vi "emi_Text from App Version.vi"(2 "Version Info":T1={"Name"="NA", "Major"=0, "Minor"=0, "Fix"=0, "Build"=0, "Type"=enum."Alfa", "Dev"=FALSE, "Version Name"="", "Date"=timestamp(0 s since 1904-01-01)} {"Date" format="%<%y%m%d>T"}, 5 "error in (no error)":errorcluster) -> (10 "Version Name":string, 11 "DEV Text":string, 12 "Name":string, 13 "Dev Only Version":bool, 14 "Filename string":string, 15 "Short version":string, 16 "Short version Type":string, 17 "Long version":string, 18 "Full version":string, 19 "error out":errorcluster)   [LabVIEW 2011]
uses:
  Private/emi_Version Info.ctl
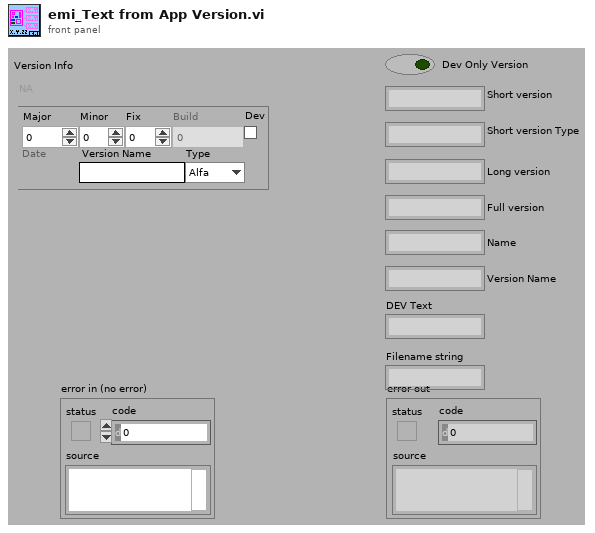
[diagram p1: front panel]
types:
  T1 = typedef "emi_Version Info.ctl" = cluster{"Name":string, "Major":i16, "Minor":i16, "Fix":i16, "Build":i32, "Type":enum16{"Alfa", "Beta", "Stable"}, "Dev":bool, "Version Name":string, "Date":timestamp}
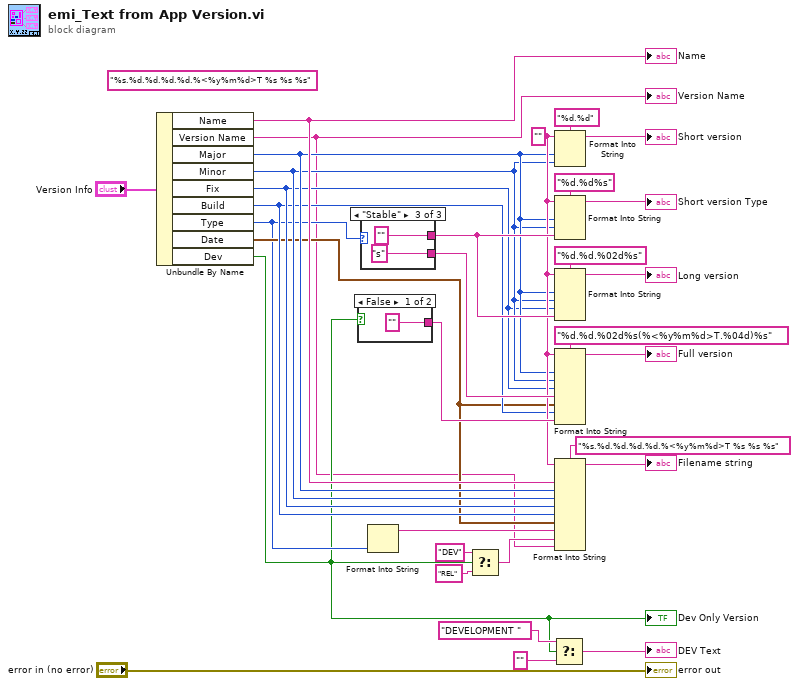
[diagram p0: block diagram]
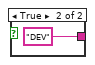
[diagram p2: hidden frame]
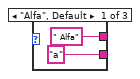
[diagram p3: hidden frame]
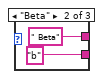
[diagram p4: hidden frame]
diagram:
  (unwired) "%s.%d.%d.%d.%d.%<%y%m%d>T %s %s %s" ("format string")
  w14 = "" ("initial string")
  n1 = Unbundle By Name("Version Info") -> ("Name"=w15:string, "Version Name"=w2:string, "Major"=w13:i16, "Minor"=w12:i16, "Fix"=w11:i16, "Build"=w10:i32, "Type"=w8:enum16{"Alfa", "Beta", "Stable"}, "Date"=w9:timestamp, "Dev"=w4:bool)
  "Dev Only Version" <- w4
  "Name" <- w15
  "Version Name" <- w2
  n2 = case shown="False" w4 {
    tunnel: ["" "DEV"] -> w29
    frame False {
      (unwired) ""
    }
    frame True {
    }
  }
  n3 = case shown="\"Stable\"" w8 {
    tunnel: [" Alfa" " Beta" ""] -> w21
    tunnel: ["a" "b" "s"] -> w27
    frame "Alfa", Default {
    }
    frame "Beta" {
    }
    frame "Stable" {
    }
  }
  n4 = Format Into String(w8) -> (resulting string=w7:string)  [unwired: 3 in, 1 out]
  n5 = Select(t="DEV" ("Version Name"), s=w4, f="REL") -> (s? t:f=w3:string)
  n6 = Select(t="DEVELOPMENT " ("Version Short"), s=w4, f="") -> (s? t:f=→"DEV Text":string)
  n7 = Format Into String(format string="%d.%d", initial string=w14, w13, w12) -> (resulting string=→"Short version":string)  [unwired: 1 in, 1 out]
  n8 = Format Into String(format string="%d.%d%s", initial string=w14, w13, w12, w21) -> (resulting string=→"Short version Type":string)  [unwired: 1 in, 1 out]
  n9 = Format Into String(format string="%d.%d.%02d%s", initial string=w14, w13, w12, w11, w21) -> (resulting string=→"Long version":string)  [unwired: 1 in, 1 out]
  n10 = Format Into String(format string="%d.%d.%02d%s(%<%y%m%d>T.%04d)%s", initial string=w14, w13, w12, w11, w27, w9, w10, w29) -> (resulting string=→"Full version":string)  [unwired: 1 in, 1 out]
  n11 = Format Into String(format string="%s.%d.%d.%d.%d.%<%y%m%d>T %s %s %s", initial string=w14, w15, w13, w12, w11, w10, w9, w7, w3, w2) -> (resulting string=→"Filename string":string)  [unwired: 1 in, 1 out]
  "error out" <- "error in (no error)"
